vi "Set Error Status.vi"(10 "status (T)":bool=TRUE, 11 "error in":errorcluster) -> (3 "error out":errorcluster)   [LabVIEW 2017, in "Memory Manager.lvlib" / "Deterministic Error Builder.lvlib"]
doc: "Sets the error status of <b>error in</b>."
uses:
  Deterministic Error Builder.lvlib
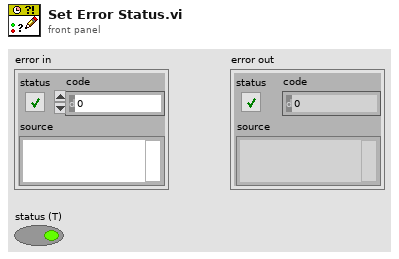
[diagram p1: front panel]
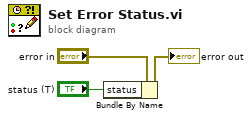
[diagram p0: block diagram]
diagram:
  n1 = Bundle By Name(cluster="error in", "status"="status (T)") -> (→"error out":errorcluster)
